vi "get images.vi"(8 "error in (no error)":errorcluster, 11 "RoomWithABomb in":refnum<class "RoomWithABomb.lvclass">) -> (0 "error out":errorcluster, 2 "images":T1[](array[typedef]), 3 "RoomWithABomb out":refnum<class "RoomWithABomb.lvclass">)   [LabVIEW 2016, in "RoomWithABomb.lvclass"]
uses:
  RoomWithABomb.lvclass
  C:/github/LVOOP-creational-patterns/Maze-Classes/src/Base/Room/Room.lvclass
  <vilib>/picture/picture.llb/imagedata.ctl
  Base/Room/Room.lvclass
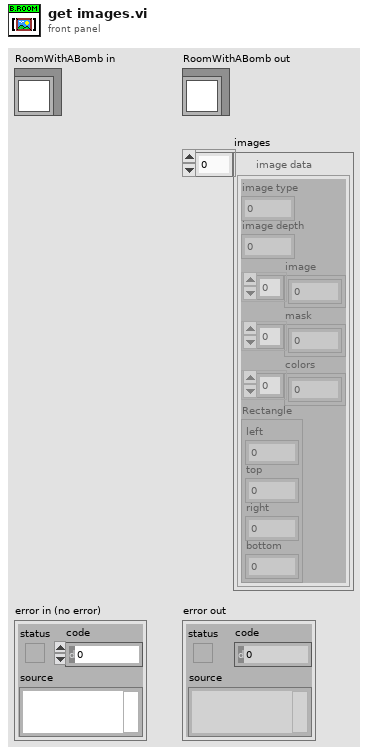
[diagram p1: front panel]
types:
  T1 = typedef "imagedata.ctl" = cluster{"image type":i32, "image depth":i32, "image":u8[], "mask":u8[], "colors":u32[], "Rectangle":cluster{"left":i16, "top":i16, "right":i16, "bottom":i16}}
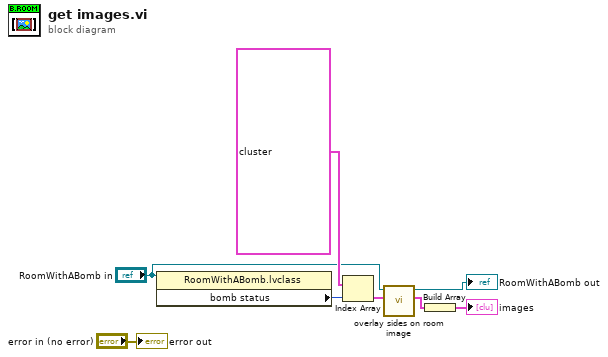
[diagram p0: block diagram]
diagram:
  n1 = property class="RoomWithABomb.lvclass"(reference="RoomWithABomb in") -> ("bomb status"=w6:enum16{"none", "exploded", "unexploded"})  [unwired: 1 in, 2 out]
  n2 = Index Array(array=T1[] [{"image type"=0, "image depth"=24, "image"=array[27648 elements], "mask"=[], "colors"=[], "Rectangle"={"left"=0, "top"=0, "right"=96, "bottom"=96}}, {"image type"=0, "image depth"=32, "image"=array[36864 elements], "mask"=array[1152 elements], "colors"=[], "Rectangle"={"left"=0, "top"=0, "right"=96, "bottom"=96}}, {"image type"=0, "image depth"=32, "image"=array[36864 elements], "mask"=array[1152 elements], "colors"=[], "Rectangle"={"left"=0, "top"=0, "right"=96, "bottom"=96}}] ("images"), index=w6) -> (element=w4:T1)
  n3 = call "overlay sides on room image.vi"("image data in"=w4, "Room in"="RoomWithABomb in") -> ("image data  out"=w1:T1, "Room out"=→"RoomWithABomb out":refnum<class "RoomWithABomb.lvclass">)  [unwired: 7 in, 1 out]
  n4 = Build Array(w1) -> (→"images":T1[])
  "error out" <- "error in (no error)"
